vi "HT3_ImgHeaderToIntArray.vi"(11 "Image Header":T1) -> (3 "Array":i32[](array[numeric]))   [LabVIEW 2009]
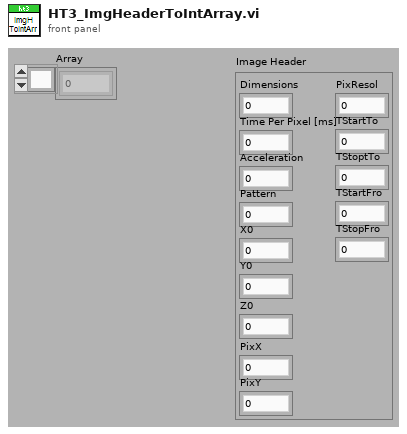
[diagram p1: front panel]
types:
  T1 = cluster{"Dimensions":i32, "Time Per Pixel [ms]":dbl, "Acceleration":i32, "Pattern":i32, "X0":sgl, "Y0":sgl, "Z0":dbl, "PixX":i32, "PixY":i32, "PixResol":sgl, "TStartTo":sgl, "TStoptTo":sgl, "TStartFro":sgl, "TStopFro":sgl}
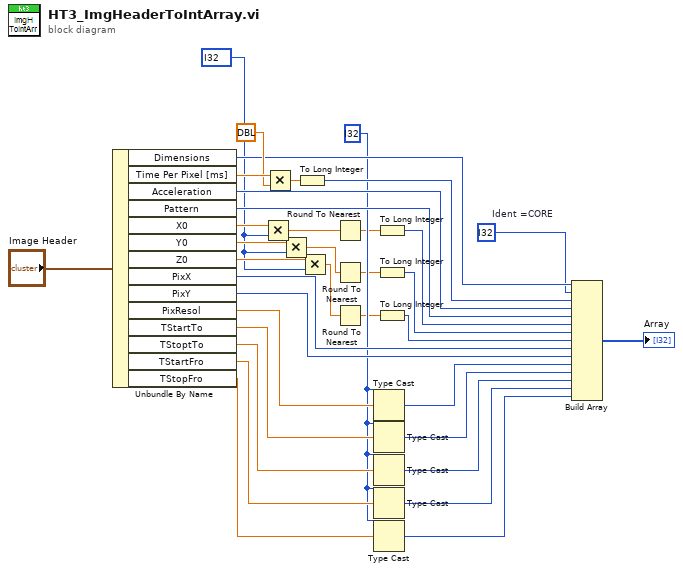
[diagram p0: block diagram]
diagram:
  w9 = i32 ?
  w24 = i32 ?  # Ident =CORE
  w12 = i32 ?
  n1 = Unbundle By Name("Image Header") -> ("Dimensions"=w25:i32, "Time Per Pixel [ms]"=w35:dbl, "Acceleration"=w22:i32, "Pattern"=w21:i32, "X0"=w13:sgl, "Y0"=w10:sgl, "Z0"=w32:dbl, "PixX"=w19:i32, "PixY"=w20:i32, "PixResol"=w28:sgl, "TStartTo"=w27:sgl, "TStoptTo"=w30:sgl, "TStartFro"=w29:sgl, "TStopFro"=w31:sgl)
  n2 = Multiply(x=w13, y=w9) -> (x*y=w11:sgl)
  n3 = Multiply(x=w35, y=dbl ?) -> (x*y=w33:dbl)
  n4 = Multiply(x=w10, y=w9) -> (x*y=w7:sgl)
  n5 = To Long Integer(number=w33) -> (32bit integer=w23:i32)
  n6 = Multiply(x=w32, y=w9) -> (x*y=w6:dbl)
  n7 = Round To Nearest(number=w11) -> (nearest integer value=w5:sgl)
  n8 = Round To Nearest(number=w7) -> (nearest integer value=w4:sgl)
  n9 = Round To Nearest(number=w6) -> (nearest integer value=w3:dbl)
  n10 = Type Cast(type=w12, x=w28) -> (*(type *) &x=w17:i32)
  n11 = Type Cast(type=w12, x=w27) -> (*(type *) &x=w16:i32)
  n12 = Type Cast(type=w12, x=w30) -> (*(type *) &x=w15:i32)
  n13 = Type Cast(type=w12, x=w29) -> (*(type *) &x=w14:i32)
  n14 = Type Cast(type=w12, x=w31) -> (*(type *) &x=w18:i32)
  n15 = To Long Integer(number=w5) -> (32bit integer=w8:i32)
  n16 = To Long Integer(number=w4) -> (32bit integer=w2:i32)
  n17 = To Long Integer(number=w3) -> (32bit integer=w1:i32)
  n18 = Build Array(w25, w24, w23, w22, w21, w8, w2, w1, w19, w20, w17, w16, w15, w14, w18) -> (→"Array":i32[])
